vi "Avrg_minute_hour_day.vi"(0 "MCU addresses":T2="B", 5 "Data ID Nr":T1 items=["", "", "", "", "", "MCU ADRESS", "", "", "", "", "ACC X", "ACC Y", "ACC Z", "ACC LEN", "TIME HOURS", "TIME MINUTS", "TIME SECONDS", "ZIGBEE TEMP", "INSIDE TEMP", "OUTSIDE TEMP", "POT111", "PIR SENSOR", "LIGHT SENSOR", "", "", "DOOR STAUS_1", "DOOR STAUS_1", "", "", "", "Empty", "Empty", "Empty", "", "", "", "", "", "", "", "", "", "", "", "", "", "", "", "", "", "", "", "", "", "", "", "", "", "", "", "", "Empty"]) -> (4 "Average over a minute":dbl, 6 "Average over an hour":dbl, 8 "Average over a day":dbl, 10 "Max Value":dbl, 15 "Min Value":dbl)   [LabVIEW 2016]
uses:
  Typedef/MCU_addresses.ctl
  Typedef/Data_ID.ctl
  <vilib>/Utility/file.llb/Read Delimited Spreadsheet (DBL).vi
panel:
  out "nearest integer value 4":dbl
  out "nearest integer value 3":dbl
  out "size(s)":i32[](array[numeric])
  out "path":path
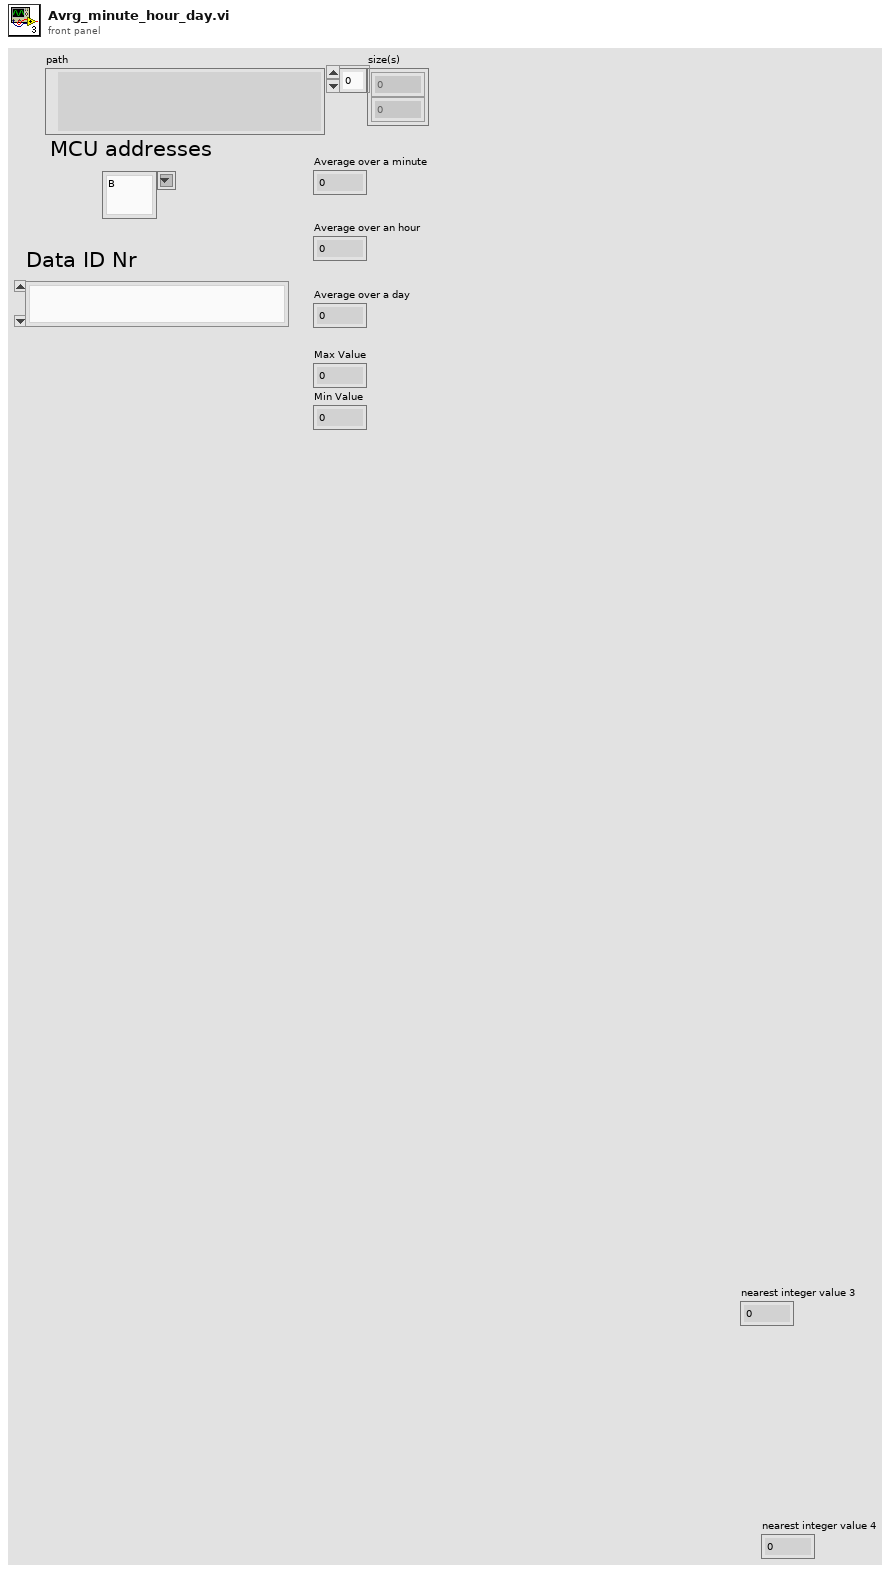
[diagram p1: front panel]
types:
  T1 = typedef "Data_ID.ctl" = u16
  T2 = typedef "MCU_addresses.ctl" = string
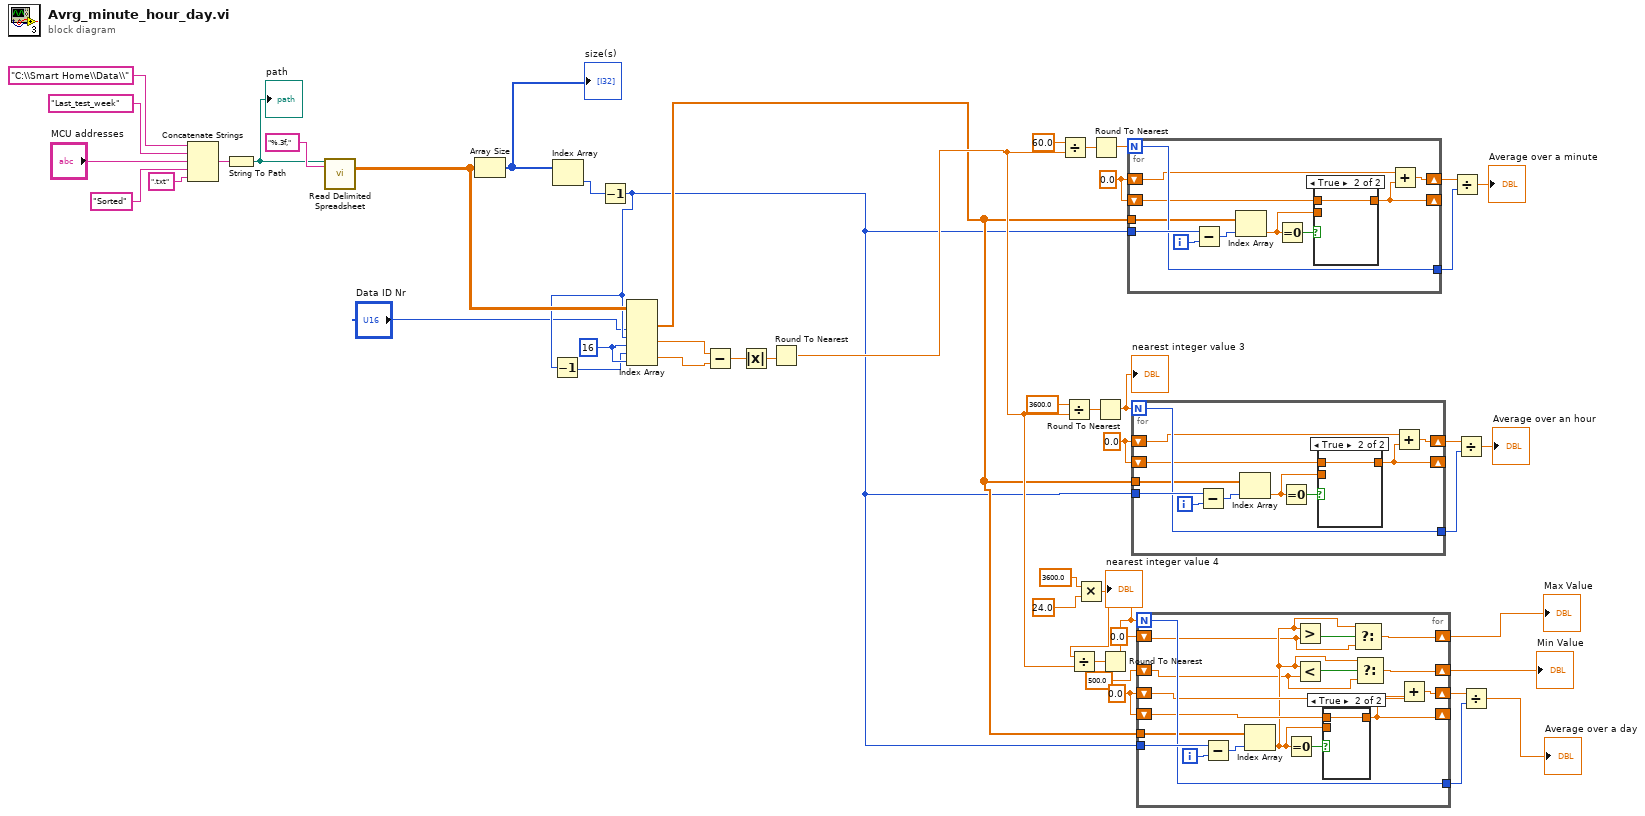
[diagram p0: block diagram]
diagram:
  w1 = 0.0 ("Numeric")
  w3 = 0.0 ("Numeric")
  w2 = 0.0 ("Numeric")
  w38 = 16 ("index (col)")
  n1 = Concatenate Strings("C:\\Smart Home\\Data\\", "Last_test_week" ("String"), "MCU addresses", "Sorted" ("string"), ".txt") -> (w48:string)
  n2 = String To Path(string=w48) -> (path=w41:path)
  "path" <- w41
  n3 = call-poly <vilib>:"Read Delimited Spreadsheet.vi"("file path (dialog if empty)"=w41, "format (%.3f)"="%.3f,") -> ("all rows"=w40:dbl[][])  [unwired: 8 in, 5 out]
  n4 = Array Size(array=w40) -> (size(s)=w39:i32[])
  "size(s)" <- w39
  n5 = Index Array(array=w39) -> (element=w36:i32)  [unwired: 1 in]
  n6 = Decrement(x=w36) -> (x-1=w9:i32)
  n7 = Decrement(x=w9) -> (x-1=w37:i32)
  n8 = Index Array(array=w40, index (col) #1="Data ID Nr", index (row) #2=w9, index (col) #2=w38, index (row) #3=w37, index (col) #3=w38) -> (element #1=w10:dbl[], element #2=w35:dbl, element #3=w34:dbl)  [unwired: 1 in]
  n9 = Subtract(x=w35, y=w34) -> (x-y=w33:dbl)
  n10 = Absolute Value(x=w33) -> (abs(x)=w32:dbl)
  n11 = Round To Nearest(number=w32) -> (nearest integer value=w14:dbl)
  n12 = Divide(x=60.0, y=w14) -> (x/y=w28:dbl)
  n13 = Divide(x=3600.0, y=w14) -> (x/y=w22:dbl)
  n14 = Multiply(x=3600.0, y=24.0) -> (x*y=w11:dbl)
  n15 = Divide(x=w11, y=w14) -> (x/y=w16:dbl)
  n16 = Round To Nearest(number=w28) -> (nearest integer value=w27:dbl)
  n17 = Round To Nearest(number=w22) -> (nearest integer value=w21:dbl)
  "nearest integer value 3" <- w21
  n18 = Round To Nearest(number=w16) -> (nearest integer value=w15:dbl)
  "nearest integer value 4" <- w15
  n19 = for {
    N: w27 -> [w55]
    tunnel: w9 -> [w57]
    shift-right: [w56] -> w30
    shift-left: w2 -> [w52]
    tunnel: [w55] -> w31
    tunnel: w10 -> [w54]
    shift-right: [w50] -> _
    shift-left: w2 -> [w49]
    i -> [w58]
    n20 = Subtract(x=w57, y=w58) -> (x-y=w59:i32)
    n21 = Index Array(array=w54, index=w59) -> (element=w51:dbl)
    n22 = Equal To 0?(x=w51) -> (x = 0?=w53:bool)
    n23 = case shown="True" w53 {
      tunnel: [w60 w61] -> w50
      tunnel: w51 -> [w60 _]
      tunnel: w49 -> [_ w61]
      frame False {
      }
      frame True {
      }
    }
    n24 = Add(x=w52, y=w50) -> (x+y=w56:dbl)
  }
  n25 = for {
    N: w21 -> [w68]
    tunnel: w9 -> [w70]
    shift-right: [w69] -> w24
    shift-left: w3 -> [w65]
    tunnel: [w68] -> w25
    tunnel: w10 -> [w67]
    shift-right: [w63] -> _
    shift-left: w3 -> [w62]
    i -> [w71]
    n26 = Subtract(x=w70, y=w71) -> (x-y=w72:i32)
    n27 = Index Array(array=w67, index=w72) -> (element=w64:dbl)
    n28 = Equal To 0?(x=w64) -> (x = 0?=w66:bool)
    n29 = case shown="True" w66 {
      tunnel: [w73 w74] -> w63
      tunnel: w64 -> [w73 _]
      tunnel: w62 -> [_ w74]
      frame False {
      }
      frame True {
      }
    }
    n30 = Add(x=w65, y=w63) -> (x+y=w69:dbl)
  }
  n31 = for {
    N: w15 -> [w87]
    tunnel: w9 -> [w89]
    shift-right: [w88] -> w18
    shift-left: w1 -> [w81]
    tunnel: [w87] -> w19
    tunnel: w10 -> [w86]
    shift-right: [w80] -> _
    shift-left: w1 -> [w84]
    shift-right: [w78] -> w7
    shift-left: 0.0 ("Numeric") -> [w75]
    shift-right: [w79] -> w6
    shift-left: 500.0 ("Numeric") -> [w76]
    i -> [w90]
    n32 = Subtract(x=w89, y=w90) -> (x-y=w91:i32)
    n33 = Index Array(array=w86, index=w91) -> (element=w77:dbl)
    n34 = Equal To 0?(x=w77) -> (x = 0?=w85:bool)
    n35 = Greater?(x=w77, y=w75) -> (0:w83:bool)
    n36 = Less?(x=w77, y=w76) -> (x < y?=w82:bool)
    n37 = case shown="True" w85 {
      tunnel: [w92 w93] -> w80
      tunnel: w77 -> [w92 _]
      tunnel: w84 -> [_ w93]
      frame False {
      }
      frame True {
      }
    }
    n38 = Select(t=w77, s=w83, f=w75) -> (s? t:f=w78:dbl)
    n39 = Select(t=w77, s=w82, f=w76) -> (s? t:f=w79:dbl)
    n40 = Add(x=w81, y=w80) -> (x+y=w88:dbl)
  }
  "Max Value" <- w7
  "Min Value" <- w6
  n41 = Divide(x=w30, y=w31) -> (x/y=→"Average over a minute":dbl)
  n42 = Divide(x=w24, y=w25) -> (x/y=→"Average over an hour":dbl)
  n43 = Divide(x=w18, y=w19) -> (x/y=→"Average over a day":dbl)
